vi "一体站流程质控自动启动.vi"(6 "CODMn量程切换":enum32{"H", "L", "AUTO"}(ring)=enum."AUTO", 8 "总磷量程切换":enum32{"H", "L", "AUTO"}(ring)=enum."AUTO", 9 "总氮量程切换":enum32{"H", "L", "AUTO"}(ring)=enum."AUTO", 10 "氨氮量程切换":enum32{"H", "L", "AUTO"}(ring)=enum."AUTO", 11 "参数":T1={"是否启用仪器"=FALSE, "CODMn"={"启动测量模式"={"测量模式"=enum."水样测量"}, "确定按钮"=TRUE}, "启动模块"={"氨氮"=FALSE, "总磷"=FALSE, "总氮"=FALSE, "CODMn"=FALSE, "CODCr"=FALSE}, "常规启动"=FALSE, "直接启动"=FALSE}) -> ()   [LabVIEW 2016, in "质控单元.lvlib"]
panel:
  out "枚举 2":enum16{"初始化", "采配水启动", "等待", "配水", "排水", "结束"}(ring)
  out "枚举":enum16{"初始化", "采配水启动", "等待", "配水", "排水", "结束"}(ring)
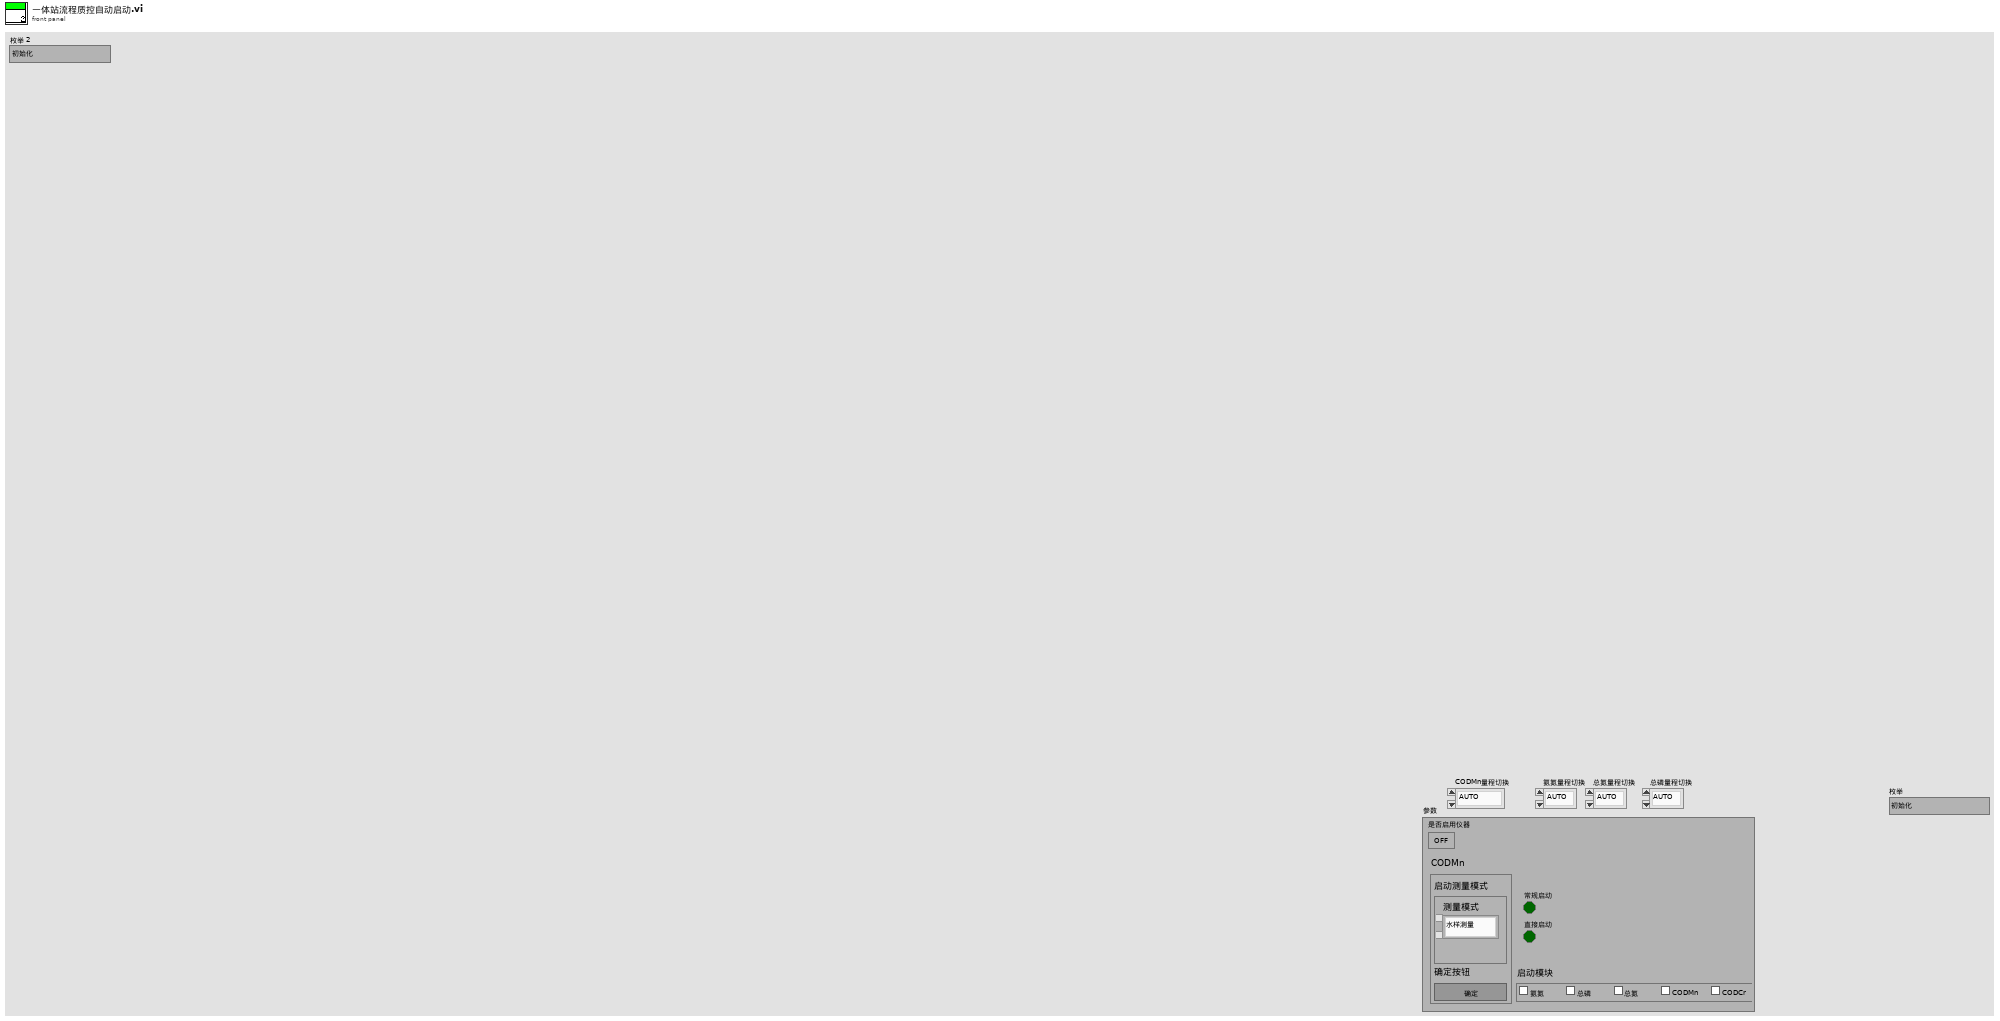
[diagram p1: front panel]
types:
  T1 = cluster{"是否启用仪器":bool, "CODMn":cluster{"启动测量模式":cluster{"测量模式":enum16{"水样测量", "标样核查", "加标回收", "平行样", "校零", "校标"}}, "确定按钮":bool}, "启动模块":cluster{"氨氮":bool, "总磷":bool, "总氮":bool, "CODMn":bool, "CODCr":bool}, "常规启动":bool, "直接启动":bool}
  T2 = cluster{"命令":string, cluster{"starting address":u16, "holding register value":u16}}
  T3 = cluster{"R0":i16, "R1":i16, "R2":i16, "R3":i16, "R4":i16, "R5":i16, "R6":i16, "R7":i16, "R8":i16, "R9":i16, "R10":i16, "R11":i16, "R12":i16, "R13":i16, "R14":i16, "R15":i16, "R16":i16, "R17":i16, "R18":i16, "R19":i16, "R20":i16, "R21":i16, "R22":i16, "R23":i16, "R24":i16, "R25":i16, "R26":i16, "R27":i16, "R28":i16, "R29":i16, "R30":i16, "R31":i16, "R32":i16, "R33":i16, "R34":i16, "R35":i16, "R36":i16, "R37":i16, "R38":i16, "R39":i16, "R40":i16, "R41":i16, "R42":i16, "R43":i16, "R44":i16, "R45":i16, "R46":i16, "R47":i16, "R48":i16, "R49":i16, "R50":i16, "R51":i16, "R52":i16, "R53":i16, "R54":i16, "R55":i16, "R56":i16}
  T4 = enum32{"Bad", "Idle", "Run top level", "Running"}
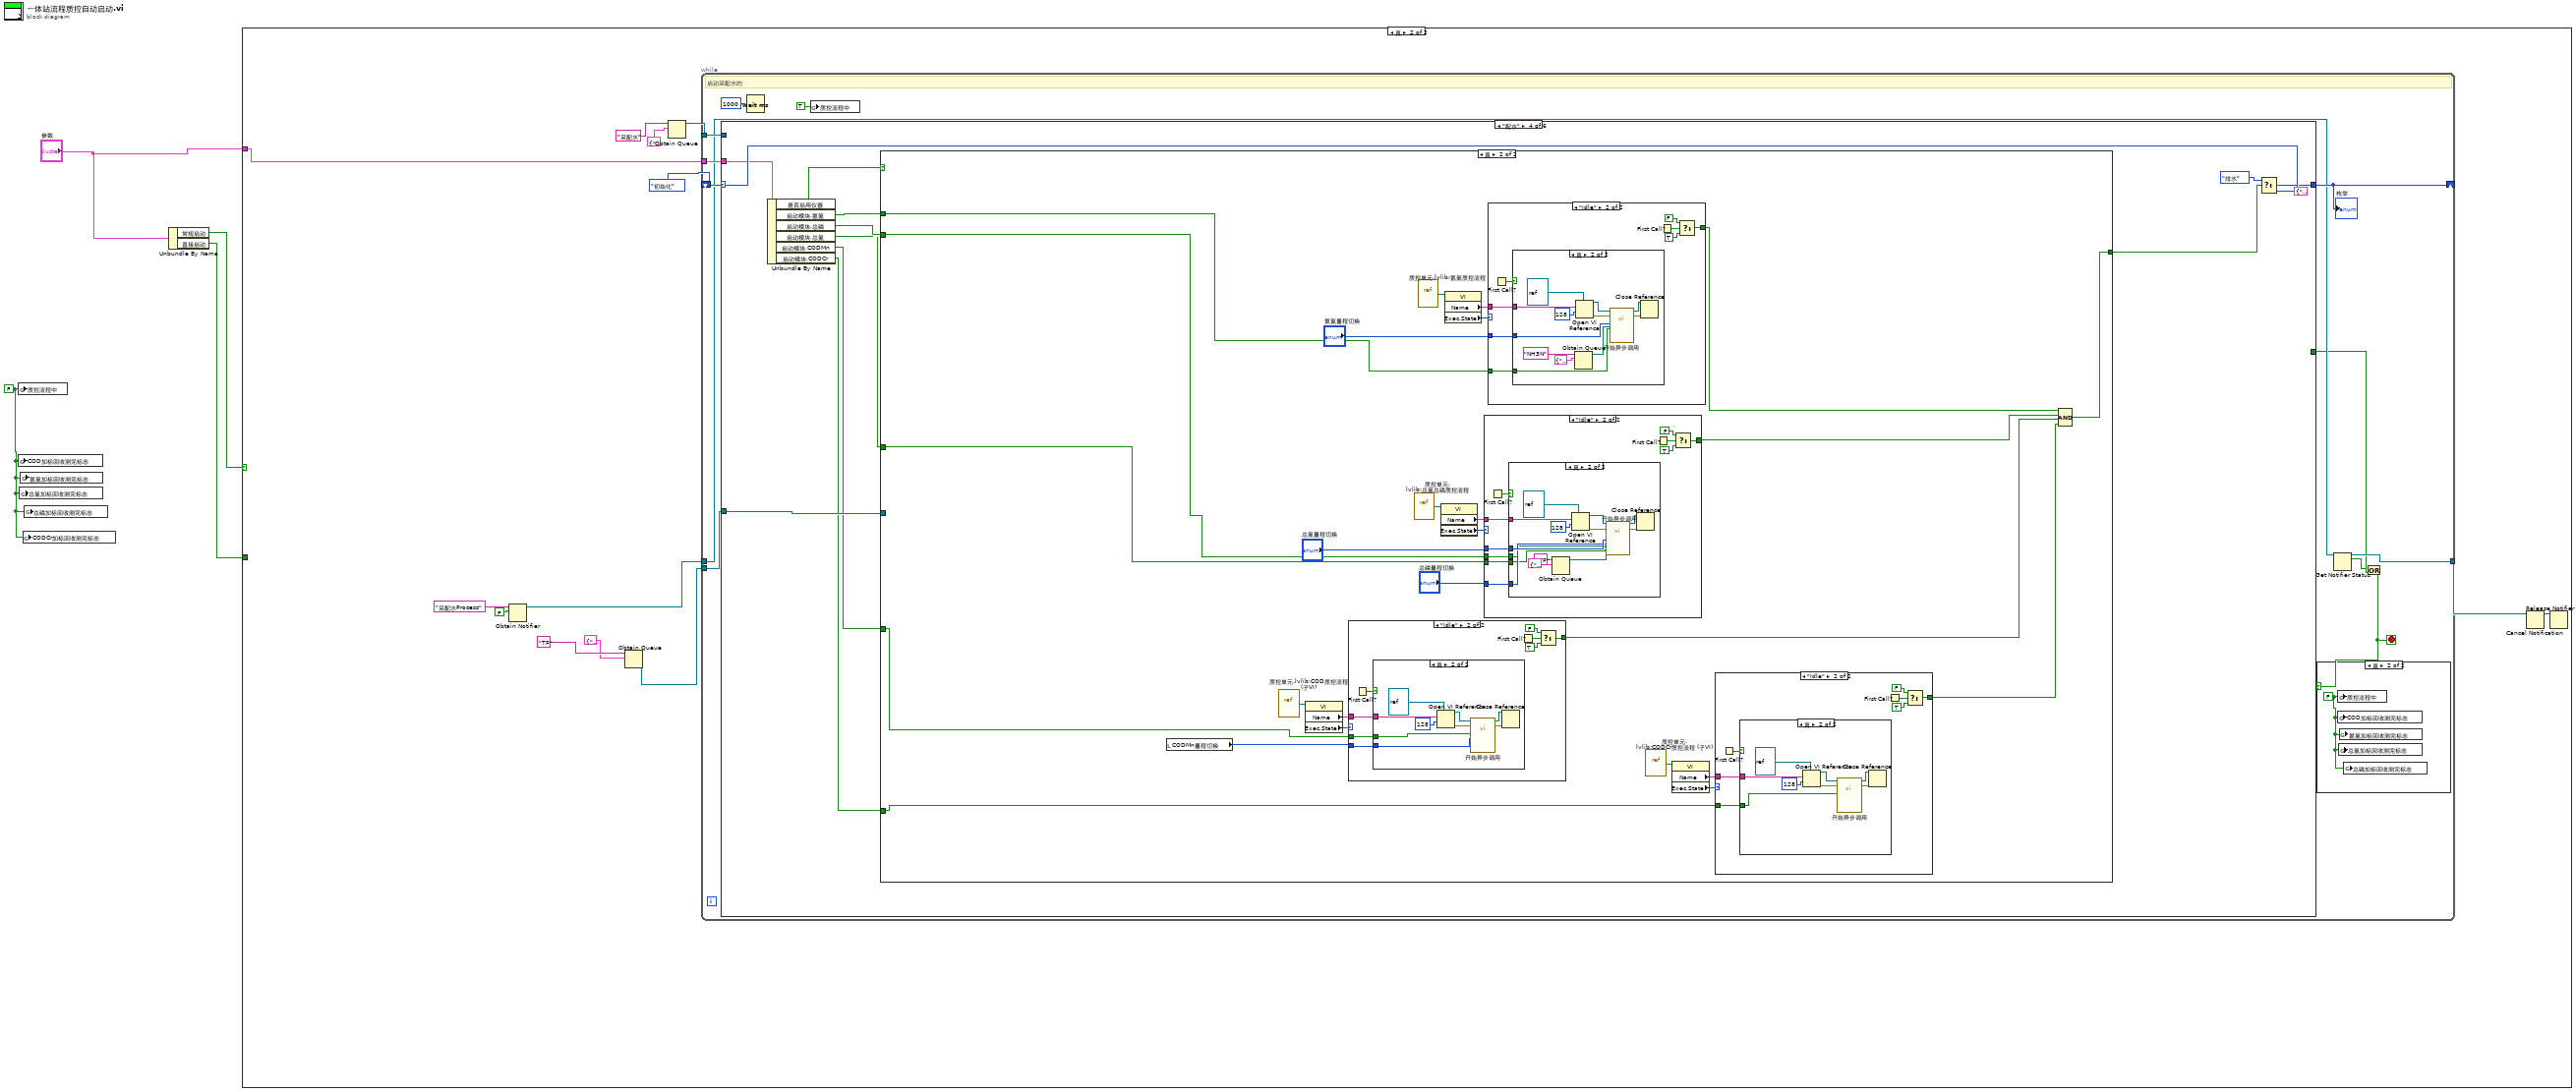
[diagram p0: block diagram]
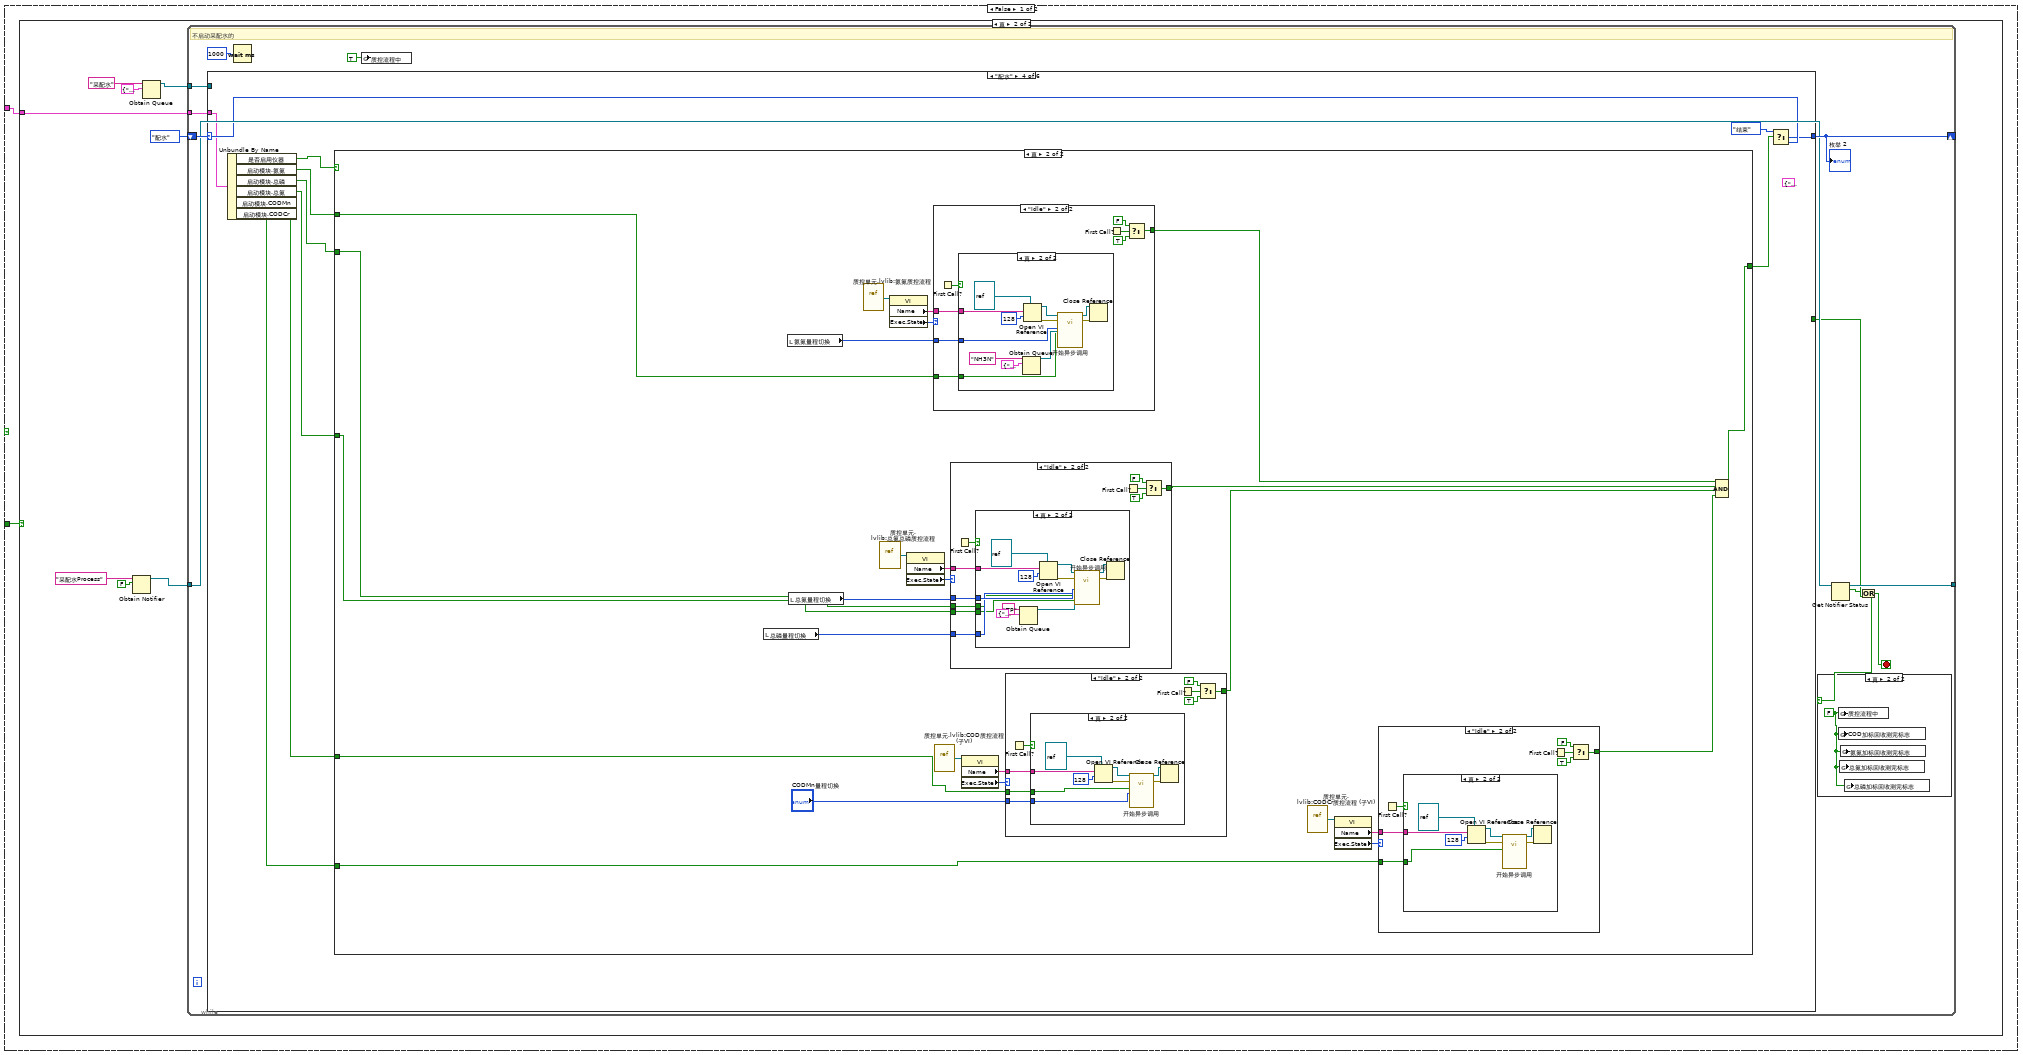
[diagram p2: hidden frame]
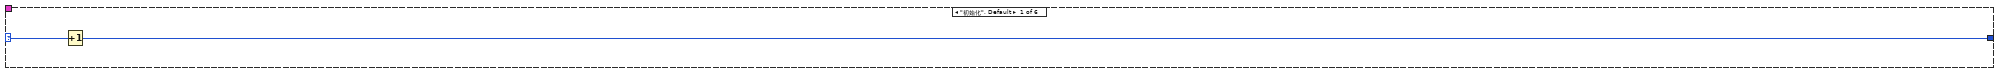
[diagram p5: hidden frame]
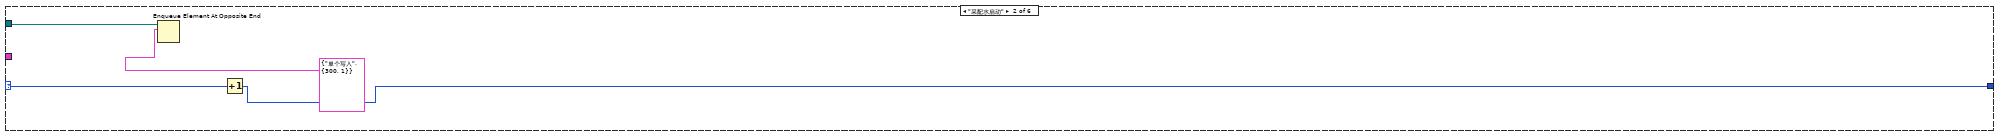
[diagram p6: hidden frame]
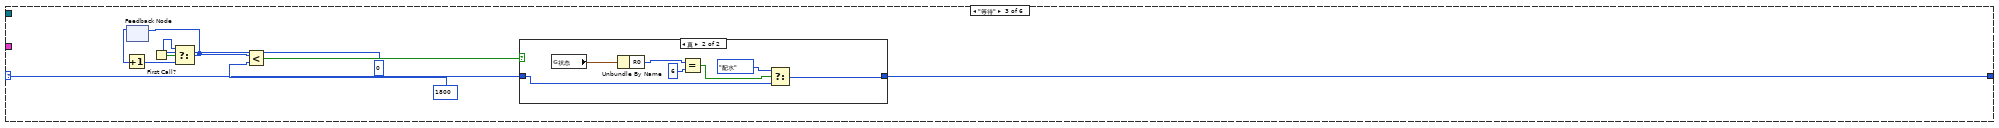
[diagram p7: hidden frame]
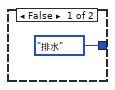
[diagram p8: hidden frame]
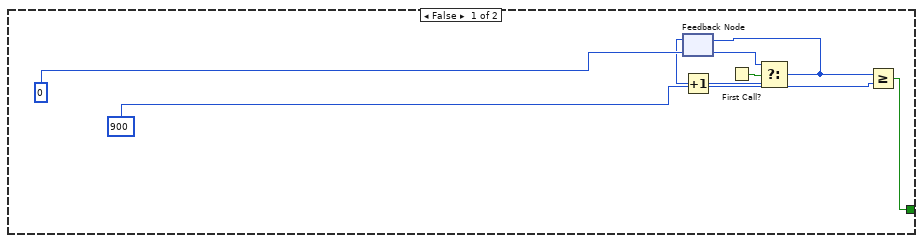
[diagram p9: hidden frame]
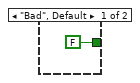
[diagram p10: hidden frame]
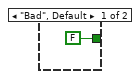
[diagram p12: hidden frame]
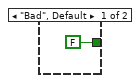
[diagram p14: hidden frame]
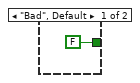
[diagram p16: hidden frame]
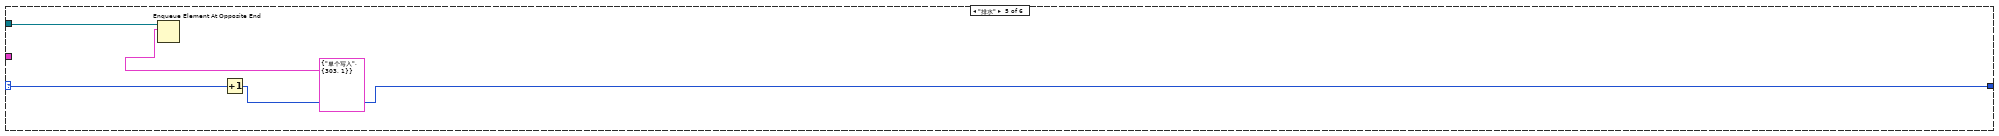
[diagram p18: hidden frame]
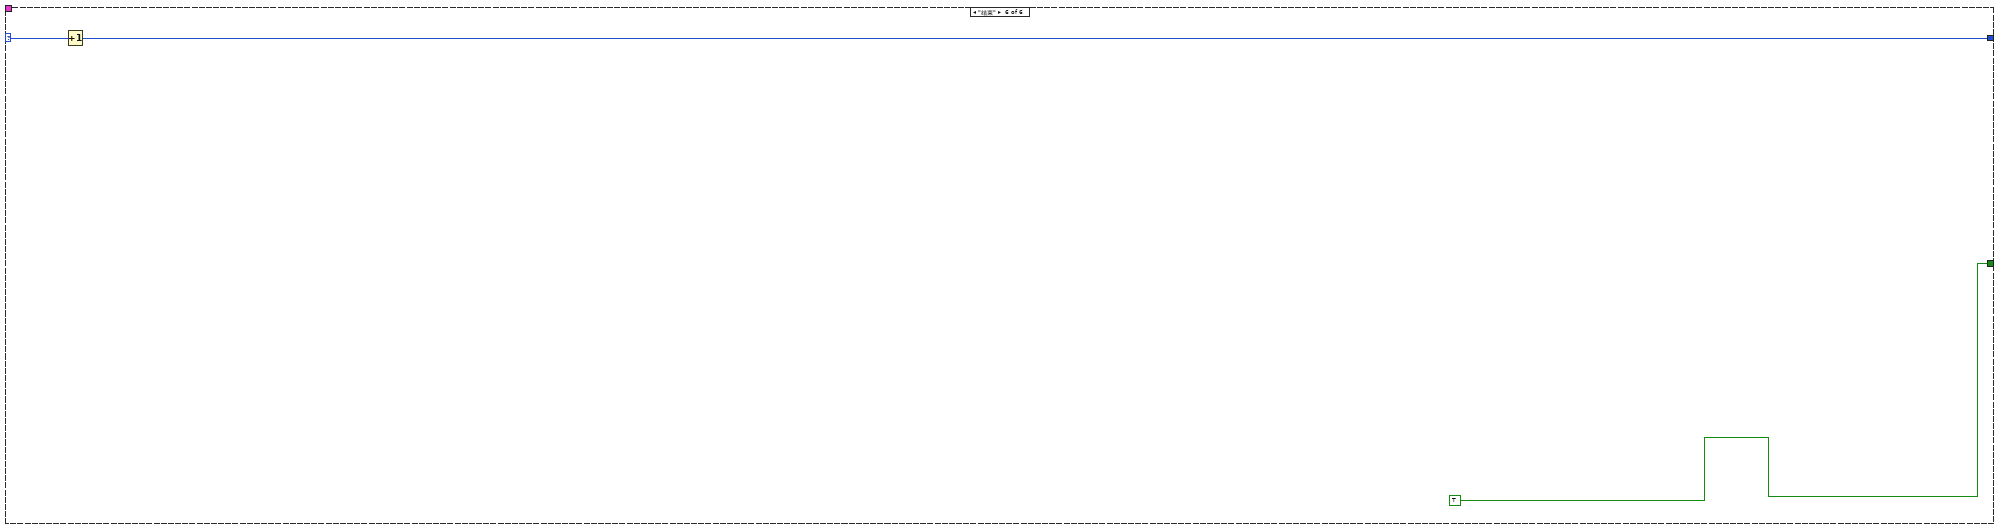
[diagram p19: hidden frame]
diagram:
  w1 = FALSE ("质控流程中")
  n1 = global write "质控测完标志全局 1.vi" "质控流程中"(w1) -> ()
  n2 = global write "质控测完标志全局 1.vi" "COD加标回收测完标志"(w1) -> ()
  n3 = global write "质控测完标志全局 1.vi" "总氮加标回收测完标志"(w1) -> ()
  n4 = global write "质控测完标志全局 1.vi" "氨氮加标回收测完标志"(w1) -> ()
  n5 = global write "质控测完标志全局 1.vi" "CODCr加标回收测完标志"(w1) -> ()
  n6 = global write "质控测完标志全局 1.vi" "总磷加标回收测完标志"(w1) -> ()
  n7 = Unbundle By Name("参数") -> ("常规启动"=w3:bool, "直接启动"=w2:bool)
  n8 = case shown="真" w3 {
    tunnel: "参数" -> [w5 w181]
    tunnel: w2 -> [w6 _]
    frame False {
      n9 = case shown="真" w6 {
        tunnel: w5 -> [_ w13]
        frame False {
        }
        frame True {
          n10 = Obtain Notifier(name (unnamed)="采配水Process" ("名称（未命名）"), notification data type=FALSE) -> (notifier out=w7:refnum<notifier>)  [unwired: 2 in, 2 out]
          n11 = Obtain Queue(name (unnamed)="采配水" ("名称（未命名）"), element data type=cluster{"命令":string, "数据":variant} {"命令"="", "数据"=variant}) -> (queue out=w10:refnum<queue>)  [unwired: 3 in, 2 out]
          n12 = while {
            tunnel: w10 -> [w25]
            shift-right: [w23] -> _
            shift-left: enum16{"初始化", "采配水启动", "等待", "配水", "排水", "结束"}."配水" ("枚举") -> [w24]
            tunnel: w13 -> [w21]
            tunnel: w7 -> [w20]
            tunnel: [w19] -> _
            stop <- w16 stop-if-true
            # "不启动采配水的"
            n13 = case shown="\"配水\"" w24 {
              selector: w24 -> [w28 w30 w39 w59 w175 w180]
              tunnel: w25 -> [_ w31 _ _ w176 _]
              tunnel: [w27 w29 w38 w58 w174 w179] -> w23
              tunnel: [_ _ _ _ _ TRUE] -> w18
              tunnel: w21 -> [_ _ _ w55 _ _]
              frame "初始化", Default {
                n14 = Increment(x=w28) -> (x+1=w27:enum16{"初始化", "采配水启动", "等待", "配水", "排水", "结束"})
              }
              frame "采配水启动" {
                n15 = Enqueue Element At Opposite End(queue=w31, element=T2 {"命令"="单个写入", {"starting address"=300, "holding register value"=1}} ("元素")) -> ()  [unwired: 2 in, 3 out]
                n16 = Increment(x=w30) -> (x+1=w29:enum16{"初始化", "采配水启动", "等待", "配水", "排水", "结束"})
              }
              frame "等待" {
                n17 = feedback #1() -> (w35:i32)  [unwired: 1 in]
                n18 = Increment(x=w35) -> (x+1=w34:i32)
                n19 = First Call?() -> (First Call?: T/F=w36:bool)
                n20 = Select(t=0, s=w36, f=w34) -> (s? t:f=w33:i32)
                n21 = feedback-in #1(w33) -> ()
                n22 = Less?(x=w33, y=1800) -> (x < y?=w40:bool)
                n23 = case shown="真" w40 {
                  tunnel: w39 -> [_ w45]
                  tunnel: [enum16{"初始化", "采配水启动", "等待", "配水", "排水", "结束"}."排水" ("枚举") w44] -> w38
                  frame False {
                  }
                  frame True {
                    n24 = global read "与采配水交互全局.vi" "状态"() -> (w43:T3)
                    n25 = Unbundle By Name(w43) -> ("R0"=w49:i16)
                    n26 = Equal?(x=w49, y=i16 6) -> (x = y?=w47:bool)
                    n27 = Select(t=enum16{"初始化", "采配水启动", "等待", "配水", "排水", "结束"}."配水" ("枚举"), s=w47, f=w45) -> (s? t:f=w44:enum16{"初始化", "采配水启动", "等待", "配水", "排水", "结束"})
                  }
                }
              }
              frame "配水" {
                (unwired) cluster{"命令":string, "data":variant} {"命令"="启动", "data"=variant(cluster{"站号":u16, "控制命令输出":u16[]} {"站号"=1, "控制命令输出"=[256, 0]})} ("元素")
                n28 = Unbundle By Name(w55) -> ("是否启用仪器"=w57:bool, "启动模块.氨氮"=w53:bool, "启动模块.总磷"=w54:bool, "启动模块.总氮"=w51:bool, "启动模块.CODMn"=w52:bool, "启动模块.CODCr"=w50:bool)
                n29 = case shown="真" w57 {
                  tunnel: [w61 w93] -> w56
                  tunnel: w54 -> [_ w81]
                  tunnel: w53 -> [_ w89]
                  tunnel: w52 -> [_ w72]
                  tunnel: w51 -> [_ w80]
                  tunnel: w50 -> [_ w69]
                  frame False {
                    n30 = feedback #2() -> (w65:i32)  [unwired: 1 in]
                    n31 = Increment(x=w65) -> (x+1=w64:i32)
                    n32 = First Call?() -> (First Call?: T/F=w66:bool)
                    n33 = Select(t=0, s=w66, f=w64) -> (s? t:f=w62:i32)
                    n34 = feedback-in #2(w62) -> ()
                    n35 = Greater Or Equal?(x=w62, y=900) -> (x >= y?=w61:bool)
                  }
                  frame True {
                    n36 = local read "总磷量程切换"() -> (w82:enum32{"H", "L", "AUTO"})
                    n37 = local read "氨氮量程切换"() -> (w87:enum32{"H", "L", "AUTO"})
                    n38 = local read "总氮量程切换"() -> (w83:enum32{"H", "L", "AUTO"})
                    n39 = vi-ref "质控单元.lvlib:氨氮质控流程.vi"() -> (w91:refnum<vi>)
                    n40 = vi-ref "质控单元.lvlib:总氮总磷质控流程.vi"() -> (w85:refnum<vi>)
                    n41 = property class="VI"(reference=w91) -> ("Name"=w92:string, "Exec.State"=w90:T4)  [unwired: 1 in, 2 out]
                    n42 = property class="VI"(reference=w85) -> ("Name"=w84:string, "Exec.State"=w86:T4)  [unwired: 1 in, 2 out]
                    n43 = case shown="\"Idle\"" w90 {
                      tunnel: w92 -> [_ w161]
                      tunnel: w89 -> [_ w160]
                      tunnel: [FALSE w155] -> w88
                      tunnel: w87 -> [_ w154]
                      frame "Bad", Default {
                      }
                      frame "Idle" {
                        n44 = First Call?() -> (First Call?: T/F=w159:bool)
                        n45 = case shown="真" w159 {
                          tunnel: w161 -> [_ w172]
                          tunnel: w160 -> [_ w163]
                          tunnel: w154 -> [_ w162]
                          frame False {
                          }
                          frame True {
                            n46 = Obtain Queue(name (unnamed)="NH3N" ("名称（未命名）"), element data type=cluster{"命令":string, "data":variant} {"命令"="", "data"=variant}) -> (queue out=w164:refnum<queue>)  [unwired: 3 in, 2 out]
                            n47 = Open VI Reference(type specifier VI Refnum (for type only)=refnum<vi> refnum ("类型说明符VI引用句柄（仅用于类型）"), vi path=w172, options=128 ("选项")) -> (vi reference=w173:refnum<vi>, error out=w169:errorcluster)  [unwired: 3 in]
                            n48 = call-by-ref "开始异步调用"(reference=w173, error in=w169, "队列输入NH3"=w164, "氨氮"=w163, "氨氮量程切换"=w162) -> (reference out=w171:refnum<vi>, error out=w170:errorcluster)  [unwired: 7 in, 2 out]
                            n49 = Close Reference(reference=w171, error in (no error)=w170) -> ()  [unwired: 1 out]
                          }
                        }
                        n50 = First Call?() -> (First Call?: T/F=w158:bool)
                        n51 = Select(t=FALSE, s=w158, f=TRUE) -> (s? t:f=w155:bool)
                      }
                    }
                    n52 = vi-ref "质控单元.lvlib:COD质控流程 (子VI).vi"() -> (w77:refnum<vi>)
                    n53 = case shown="\"Idle\"" w86 {
                      tunnel: w84 -> [_ w138]
                      tunnel: w82 -> [_ w137]
                      tunnel: [FALSE w132] -> w79
                      tunnel: w83 -> [_ w131]
                      tunnel: w81 -> [_ w130]
                      tunnel: w80 -> [_ w129]
                      frame "Bad", Default {
                      }
                      frame "Idle" {
                        n54 = First Call?() -> (First Call?: T/F=w136:bool)
                        n55 = case shown="真" w136 {
                          tunnel: w138 -> [_ w152]
                          tunnel: w137 -> [_ w141]
                          tunnel: w131 -> [_ w142]
                          tunnel: w130 -> [_ w140]
                          tunnel: w129 -> [_ w139]
                          frame False {
                          }
                          frame True {
                            n56 = Obtain Queue(name (unnamed)="TP" ("名称（未命名）"), element data type=cluster{"命令":string, "data":variant} {"命令"="", "data"=variant}) -> (queue out=w143:refnum<queue>)  [unwired: 3 in, 2 out]
                            n57 = Open VI Reference(type specifier VI Refnum (for type only)=refnum<vi> refnum ("类型说明符VI引用句柄（仅用于类型）"), vi path=w152, options=128 ("选项")) -> (vi reference=w144:refnum<vi>, error out=w149:errorcluster)  [unwired: 3 in]
                            n58 = call-by-ref "开始异步调用"(reference=w144, error in=w149, "队列输入TP"=w143, "总氮量程切换"=w142, "总磷量程切换"=w141, "总磷"=w140, "总氮"=w139) -> (reference out=w151:refnum<vi>, error out=w150:errorcluster)  [unwired: 8 in, 3 out]
                            n59 = Close Reference(reference=w151, error in (no error)=w150) -> ()  [unwired: 1 out]
                          }
                        }
                        n60 = First Call?() -> (First Call?: T/F=w135:bool)
                        n61 = Select(t=FALSE, s=w135, f=TRUE) -> (s? t:f=w132:bool)
                      }
                    }
                    n62 = property class="VI"(reference=w77) -> ("Name"=w78:string, "Exec.State"=w76:T4)  [unwired: 1 in, 2 out]
                    n63 = case shown="\"Idle\"" w76 {
                      tunnel: w78 -> [_ w118]
                      tunnel: [FALSE w113] -> w70
                      tunnel: "CODMn量程切换" -> [_ w112]
                      tunnel: w72 -> [_ w111]
                      frame "Bad", Default {
                      }
                      frame "Idle" {
                        n64 = First Call?() -> (First Call?: T/F=w117:bool)
                        n65 = case shown="真" w117 {
                          tunnel: w118 -> [_ w126]
                          tunnel: w112 -> [_ w119]
                          tunnel: w111 -> [_ w120]
                          frame False {
                          }
                          frame True {
                            n66 = Open VI Reference(type specifier VI Refnum (for type only)=refnum<vi> refnum ("类型说明符VI引用句柄（仅用于类型）"), vi path=w126, options=128 ("选项")) -> (vi reference=w127:refnum<vi>, error out=w123:errorcluster)  [unwired: 3 in]
                            n67 = call-by-ref "开始异步调用"(reference=w127, error in=w123, "CODMn量程切换"=w119, "COD"=w120) -> (reference out=w125:refnum<vi>, error out=w124:errorcluster)  [unwired: 8 in, 2 out]
                            n68 = Close Reference(reference=w125, error in (no error)=w124) -> ()  [unwired: 1 out]
                          }
                        }
                        n69 = First Call?() -> (First Call?: T/F=w116:bool)
                        n70 = Select(t=FALSE, s=w116, f=TRUE) -> (s? t:f=w113:bool)
                      }
                    }
                    n71 = vi-ref "质控单元.lvlib:CODCr质控流程 (子VI).vi"() -> (w74:refnum<vi>)
                    n72 = property class="VI"(reference=w74) -> ("Name"=w75:string, "Exec.State"=w73:T4)  [unwired: 1 in, 2 out]
                    n73 = case shown="\"Idle\"" w73 {
                      tunnel: w75 -> [_ w101]
                      tunnel: [FALSE w96] -> w68
                      tunnel: w69 -> [_ w95]
                      frame "Bad", Default {
                      }
                      frame "Idle" {
                        n74 = First Call?() -> (First Call?: T/F=w100:bool)
                        n75 = case shown="真" w100 {
                          tunnel: w101 -> [_ w108]
                          tunnel: w95 -> [_ w102]
                          frame False {
                          }
                          frame True {
                            n76 = Open VI Reference(type specifier VI Refnum (for type only)=refnum<vi> refnum ("类型说明符VI引用句柄（仅用于类型）"), vi path=w108, options=128 ("选项")) -> (vi reference=w109:refnum<vi>, error out=w105:errorcluster)  [unwired: 3 in]
                            n77 = call-by-ref "开始异步调用"(reference=w109, error in=w105, "CODCr"=w102) -> (reference out=w107:refnum<vi>, error out=w106:errorcluster)  [unwired: 9 in, 2 out]
                            n78 = Close Reference(reference=w107, error in (no error)=w106) -> ()  [unwired: 1 out]
                          }
                        }
                        n79 = First Call?() -> (First Call?: T/F=w99:bool)
                        n80 = Select(t=FALSE, s=w99, f=TRUE) -> (s? t:f=w96:bool)
                      }
                    }
                    n81 = Compound Arithmetic op=AND ("复合运算")(w88, w79, w70, w68) -> (w93:bool)
                  }
                }
                n82 = Select(t=enum16{"初始化", "采配水启动", "等待", "配水", "排水", "结束"}."结束" ("枚举"), s=w56, f=w59) -> (s? t:f=w58:enum16{"初始化", "采配水启动", "等待", "配水", "排水", "结束"})
              }
              frame "排水" {
                n83 = Enqueue Element At Opposite End(queue=w176, element=T2 {"命令"="单个写入", {"starting address"=303, "holding register value"=1}} ("元素")) -> ()  [unwired: 2 in, 3 out]
                n84 = Increment(x=w175) -> (x+1=w174:enum16{"初始化", "采配水启动", "等待", "配水", "排水", "结束"})
              }
              frame "结束" {
                n85 = Increment(x=w180) -> (x+1=w179:enum16{"初始化", "采配水启动", "等待", "配水", "排水", "结束"})
              }
            }
            "枚举 2" <- w23
            n86 = Wait (ms)(milliseconds to wait=u32 1000 ("等待时间（毫秒）")) -> ()  [unwired: 1 out]
            n87 = global write "质控测完标志全局 1.vi" "质控流程中"(TRUE ("质控流程中")) -> ()
            n88 = Get Notifier Status(notifier=w20) -> (notifier out=w19:refnum<notifier>, current notification=w17:bool)  [unwired: 1 in, 3 out]
            n89 = Or(x=w17, y=w18) -> (x .or. y?=w16:bool)
            n90 = case shown="真" w16 {
              frame False {
              }
              frame True {
                w26 = FALSE ("质控流程中")
                n91 = global write "质控测完标志全局 1.vi" "质控流程中"(w26) -> ()
                n92 = global write "质控测完标志全局 1.vi" "COD加标回收测完标志"(w26) -> ()
                n93 = global write "质控测完标志全局 1.vi" "总氮加标回收测完标志"(w26) -> ()
                n94 = global write "质控测完标志全局 1.vi" "氨氮加标回收测完标志"(w26) -> ()
                n95 = global write "质控测完标志全局 1.vi" "总磷加标回收测完标志"(w26) -> ()
              }
            }
          }
        }
      }
    }
    frame True {
      n96 = Obtain Notifier(name (unnamed)="采配水Process" ("名称（未命名）"), notification data type=FALSE) -> (notifier out=w184:refnum<notifier>)  [unwired: 2 in, 2 out]
      n97 = Obtain Queue(name (unnamed)="TP" ("名称（未命名）"), element data type=cluster{"命令":string, "data":variant} {"命令"="", "data"=variant}) -> (queue out=w187:refnum<queue>)  [unwired: 3 in, 2 out]
      n98 = Obtain Queue(name (unnamed)="采配水" ("名称（未命名）"), element data type=cluster{"命令":string, "数据":variant} {"命令"="", "数据"=variant}) -> (queue out=w191:refnum<queue>)  [unwired: 3 in, 2 out]
      n99 = while {
        tunnel: w191 -> [w205]
        shift-right: [w203] -> _
        shift-left: enum16{"初始化", "采配水启动", "等待", "配水", "排水", "结束"}."初始化" ("枚举") -> [w204]
        tunnel: w187 -> [w201]
        tunnel: w181 -> [w200]
        tunnel: w184 -> [w199]
        tunnel: [w198] -> w183
        stop <- w195 stop-if-true
        # "启动采配水的"
        n100 = case shown="\"配水\"" w204 {
          selector: w204 -> [w208 w210 w219 w240 w356 w361]
          tunnel: w205 -> [_ w211 _ _ w357 _]
          tunnel: [w207 w209 w218 w239 w355 w360] -> w203
          tunnel: [_ _ _ _ _ TRUE] -> w197
          tunnel: w201 -> [_ _ _ w238 _ _]
          tunnel: w200 -> [_ _ _ w235 _ _]
          frame "初始化", Default {
            n101 = Increment(x=w208) -> (x+1=w207:enum16{"初始化", "采配水启动", "等待", "配水", "排水", "结束"})
          }
          frame "采配水启动" {
            n102 = Enqueue Element At Opposite End(queue=w211, element=T2 {"命令"="单个写入", {"starting address"=300, "holding register value"=1}} ("元素")) -> ()  [unwired: 2 in, 3 out]
            n103 = Increment(x=w210) -> (x+1=w209:enum16{"初始化", "采配水启动", "等待", "配水", "排水", "结束"})
          }
          frame "等待" {
            n104 = feedback #3() -> (w215:i32)  [unwired: 1 in]
            n105 = Increment(x=w215) -> (x+1=w214:i32)
            n106 = First Call?() -> (First Call?: T/F=w216:bool)
            n107 = Select(t=0, s=w216, f=w214) -> (s? t:f=w213:i32)
            n108 = feedback-in #3(w213) -> ()
            n109 = Less?(x=w213, y=1800) -> (x < y?=w220:bool)
            n110 = case shown="真" w220 {
              tunnel: w219 -> [_ w225]
              tunnel: [enum16{"初始化", "采配水启动", "等待", "配水", "排水", "结束"}."排水" ("枚举") w224] -> w218
              frame False {
              }
              frame True {
                n111 = global read "与采配水交互全局.vi" "状态"() -> (w223:T3)
                n112 = Unbundle By Name(w223) -> ("R0"=w229:i16)
                n113 = Equal?(x=w229, y=i16 6) -> (x = y?=w227:bool)
                n114 = Select(t=enum16{"初始化", "采配水启动", "等待", "配水", "排水", "结束"}."配水" ("枚举"), s=w227, f=w225) -> (s? t:f=w224:enum16{"初始化", "采配水启动", "等待", "配水", "排水", "结束"})
              }
            }
          }
          frame "配水" {
            (unwired) cluster{"命令":string, "data":variant} {"命令"="启动", "data"=variant(cluster{"站号":u16, "控制命令输出":u16[]} {"站号"=1, "控制命令输出"=[256, 0]})} ("元素")
            n115 = Unbundle By Name(w235) -> ("是否启用仪器"=w237:bool, "启动模块.氨氮"=w233:bool, "启动模块.总磷"=w234:bool, "启动模块.总氮"=w231:bool, "启动模块.CODMn"=w232:bool, "启动模块.CODCr"=w230:bool)
            n116 = case shown="真" w237 {
              tunnel: w238 -> [_ _]
              tunnel: [w242 w274] -> w236
              tunnel: w234 -> [_ w263]
              tunnel: w233 -> [_ w269]
              tunnel: w232 -> [_ w252]
              tunnel: w231 -> [_ w262]
              tunnel: w230 -> [_ w251]
              frame False {
                n117 = feedback #4() -> (w246:i32)  [unwired: 1 in]
                n118 = Increment(x=w246) -> (x+1=w245:i32)
                n119 = First Call?() -> (First Call?: T/F=w247:bool)
                n120 = Select(t=0, s=w247, f=w245) -> (s? t:f=w243:i32)
                n121 = feedback-in #4(w243) -> ()
                n122 = Greater Or Equal?(x=w243, y=900) -> (x >= y?=w242:bool)
              }
              frame True {
                n123 = local read "CODMn量程切换"() -> (w253:enum32{"H", "L", "AUTO"})
                n124 = vi-ref "质控单元.lvlib:COD质控流程 (子VI).vi"() -> (w258:refnum<vi>)
                n125 = property class="VI"(reference=w258) -> ("Name"=w259:string, "Exec.State"=w257:T4)  [unwired: 1 in, 2 out]
                n126 = case shown="\"Idle\"" w257 {
                  tunnel: w259 -> [_ w299]
                  tunnel: [FALSE w294] -> w250
                  tunnel: w253 -> [_ w293]
                  tunnel: w252 -> [_ w292]
                  frame "Bad", Default {
                  }
                  frame "Idle" {
                    n127 = First Call?() -> (First Call?: T/F=w298:bool)
                    n128 = case shown="真" w298 {
                      tunnel: w299 -> [_ w307]
                      tunnel: w293 -> [_ w300]
                      tunnel: w292 -> [_ w301]
                      frame False {
                      }
                      frame True {
                        n129 = Open VI Reference(type specifier VI Refnum (for type only)=refnum<vi> refnum ("类型说明符VI引用句柄（仅用于类型）"), vi path=w307, options=128 ("选项")) -> (vi reference=w308:refnum<vi>, error out=w304:errorcluster)  [unwired: 3 in]
                        n130 = call-by-ref "开始异步调用"(reference=w308, error in=w304, "CODMn量程切换"=w300, "COD"=w301) -> (reference out=w306:refnum<vi>, error out=w305:errorcluster)  [unwired: 8 in, 2 out]
                        n131 = Close Reference(reference=w306, error in (no error)=w305) -> ()  [unwired: 1 out]
                      }
                    }
                    n132 = First Call?() -> (First Call?: T/F=w297:bool)
                    n133 = Select(t=FALSE, s=w297, f=TRUE) -> (s? t:f=w294:bool)
                  }
                }
                n134 = vi-ref "质控单元.lvlib:总氮总磷质控流程.vi"() -> (w267:refnum<vi>)
                n135 = vi-ref "质控单元.lvlib:氨氮质控流程.vi"() -> (w272:refnum<vi>)
                n136 = property class="VI"(reference=w267) -> ("Name"=w266:string, "Exec.State"=w268:T4)  [unwired: 1 in, 2 out]
                n137 = property class="VI"(reference=w272) -> ("Name"=w273:string, "Exec.State"=w271:T4)  [unwired: 1 in, 2 out]
                n138 = case shown="\"Idle\"" w268 {
                  tunnel: w266 -> [_ w319]
                  tunnel: "总磷量程切换" -> [_ w318]
                  tunnel: [FALSE w313] -> w264
                  tunnel: "总氮量程切换" -> [_ w312]
                  tunnel: w263 -> [_ w311]
                  tunnel: w262 -> [_ w310]
                  frame "Bad", Default {
                  }
                  frame "Idle" {
                    n139 = First Call?() -> (First Call?: T/F=w317:bool)
                    n140 = case shown="真" w317 {
                      tunnel: w319 -> [_ w333]
                      tunnel: w318 -> [_ w322]
                      tunnel: w312 -> [_ w323]
                      tunnel: w311 -> [_ w321]
                      tunnel: w310 -> [_ w320]
                      frame False {
                      }
                      frame True {
                        n141 = Obtain Queue(name (unnamed)="TP" ("名称（未命名）"), element data type=cluster{"命令":string, "data":variant} {"命令"="", "data"=variant}) -> (queue out=w324:refnum<queue>)  [unwired: 3 in, 2 out]
                        n142 = Open VI Reference(type specifier VI Refnum (for type only)=refnum<vi> refnum ("类型说明符VI引用句柄（仅用于类型）"), vi path=w333, options=128 ("选项")) -> (vi reference=w325:refnum<vi>, error out=w330:errorcluster)  [unwired: 3 in]
                        n143 = call-by-ref "开始异步调用"(reference=w325, error in=w330, "队列输入TP"=w324, "总氮量程切换"=w323, "总磷量程切换"=w322, "总磷"=w321, "总氮"=w320) -> (reference out=w332:refnum<vi>, error out=w331:errorcluster)  [unwired: 8 in, 3 out]
                        n144 = Close Reference(reference=w332, error in (no error)=w331) -> ()  [unwired: 1 out]
                      }
                    }
                    n145 = First Call?() -> (First Call?: T/F=w316:bool)
                    n146 = Select(t=FALSE, s=w316, f=TRUE) -> (s? t:f=w313:bool)
                  }
                }
                n147 = case shown="\"Idle\"" w271 {
                  tunnel: w273 -> [_ w342]
                  tunnel: w269 -> [_ w341]
                  tunnel: [FALSE w336] -> w265
                  tunnel: "氨氮量程切换" -> [_ w335]
                  frame "Bad", Default {
                  }
                  frame "Idle" {
                    n148 = First Call?() -> (First Call?: T/F=w340:bool)
                    n149 = case shown="真" w340 {
                      tunnel: w342 -> [_ w353]
                      tunnel: w341 -> [_ w344]
                      tunnel: w335 -> [_ w343]
                      frame False {
                      }
                      frame True {
                        n150 = Obtain Queue(name (unnamed)="NH3N" ("名称（未命名）"), element data type=cluster{"命令":string, "data":variant} {"命令"="", "data"=variant}) -> (queue out=w345:refnum<queue>)  [unwired: 3 in, 2 out]
                        n151 = Open VI Reference(type specifier VI Refnum (for type only)=refnum<vi> refnum ("类型说明符VI引用句柄（仅用于类型）"), vi path=w353, options=128 ("选项")) -> (vi reference=w354:refnum<vi>, error out=w350:errorcluster)  [unwired: 3 in]
                        n152 = call-by-ref "开始异步调用"(reference=w354, error in=w350, "队列输入NH3"=w345, "氨氮"=w344, "氨氮量程切换"=w343) -> (reference out=w352:refnum<vi>, error out=w351:errorcluster)  [unwired: 7 in, 2 out]
                        n153 = Close Reference(reference=w352, error in (no error)=w351) -> ()  [unwired: 1 out]
                      }
                    }
                    n154 = First Call?() -> (First Call?: T/F=w339:bool)
                    n155 = Select(t=FALSE, s=w339, f=TRUE) -> (s? t:f=w336:bool)
                  }
                }
                n156 = vi-ref "质控单元.lvlib:CODCr质控流程 (子VI).vi"() -> (w255:refnum<vi>)
                n157 = property class="VI"(reference=w255) -> ("Name"=w256:string, "Exec.State"=w254:T4)  [unwired: 1 in, 2 out]
                n158 = case shown="\"Idle\"" w254 {
                  tunnel: w256 -> [_ w282]
                  tunnel: [FALSE w277] -> w249
                  tunnel: w251 -> [_ w276]
                  frame "Bad", Default {
                  }
                  frame "Idle" {
                    n159 = First Call?() -> (First Call?: T/F=w281:bool)
                    n160 = case shown="真" w281 {
                      tunnel: w282 -> [_ w289]
                      tunnel: w276 -> [_ w283]
                      frame False {
                      }
                      frame True {
                        n161 = Open VI Reference(type specifier VI Refnum (for type only)=refnum<vi> refnum ("类型说明符VI引用句柄（仅用于类型）"), vi path=w289, options=128 ("选项")) -> (vi reference=w290:refnum<vi>, error out=w286:errorcluster)  [unwired: 3 in]
                        n162 = call-by-ref "开始异步调用"(reference=w290, error in=w286, "CODCr"=w283) -> (reference out=w288:refnum<vi>, error out=w287:errorcluster)  [unwired: 9 in, 2 out]
                        n163 = Close Reference(reference=w288, error in (no error)=w287) -> ()  [unwired: 1 out]
                      }
                    }
                    n164 = First Call?() -> (First Call?: T/F=w280:bool)
                    n165 = Select(t=FALSE, s=w280, f=TRUE) -> (s? t:f=w277:bool)
                  }
                }
                n166 = Compound Arithmetic op=AND ("复合运算")(w265, w264, w250, w249) -> (w274:bool)
              }
            }
            n167 = Select(t=enum16{"初始化", "采配水启动", "等待", "配水", "排水", "结束"}."排水" ("枚举"), s=w236, f=w240) -> (s? t:f=w239:enum16{"初始化", "采配水启动", "等待", "配水", "排水", "结束"})
          }
          frame "排水" {
            n168 = Enqueue Element At Opposite End(queue=w357, element=T2 {"命令"="单个写入", {"starting address"=303, "holding register value"=1}} ("元素")) -> ()  [unwired: 2 in, 3 out]
            n169 = Increment(x=w356) -> (x+1=w355:enum16{"初始化", "采配水启动", "等待", "配水", "排水", "结束"})
          }
          frame "结束" {
            n170 = Increment(x=w361) -> (x+1=w360:enum16{"初始化", "采配水启动", "等待", "配水", "排水", "结束"})
          }
        }
        "枚举" <- w203
        n171 = Wait (ms)(milliseconds to wait=u32 1000 ("等待时间（毫秒）")) -> ()  [unwired: 1 out]
        n172 = global write "质控测完标志全局 1.vi" "质控流程中"(TRUE ("质控流程中")) -> ()
        n173 = Get Notifier Status(notifier=w199) -> (notifier out=w198:refnum<notifier>, current notification=w196:bool)  [unwired: 1 in, 3 out]
        n174 = Or(x=w196, y=w197) -> (x .or. y?=w195:bool)
        n175 = case shown="真" w195 {
          frame False {
          }
          frame True {
            w206 = FALSE ("质控流程中")
            n176 = global write "质控测完标志全局 1.vi" "质控流程中"(w206) -> ()
            n177 = global write "质控测完标志全局 1.vi" "COD加标回收测完标志"(w206) -> ()
            n178 = global write "质控测完标志全局 1.vi" "总氮加标回收测完标志"(w206) -> ()
            n179 = global write "质控测完标志全局 1.vi" "氨氮加标回收测完标志"(w206) -> ()
            n180 = global write "质控测完标志全局 1.vi" "总磷加标回收测完标志"(w206) -> ()
          }
        }
      }
      n181 = Cancel Notification(0:w183) -> (8:w182:refnum<notifier>)  [unwired: 1 in, 2 out]
      n182 = Release Notifier(notifier=w182) -> ()  [unwired: 2 in, 3 out]
    }
  }
